vi "zlock_sendrecv.vi"(8 "error in (no error)":errorcluster, 10 "parts":string[](array[string]), 11 "socket in":T1) -> (0 "error out":errorcluster, 2 "reply":string, 3 "socket out":T1)   [LabVIEW 2010]
uses:
  <userlib>/BIAS2/subvis/zlock/zlock.ctl
  <vilib>/addons/zeromq/zmq_context.lvclass
  <vilib>/addons/zeromq/socket_type.ctl
  <vilib>/addons/zeromq/zmq_socket.lvclass
  <vilib>/addons/zeromq/zeromq.lvlib
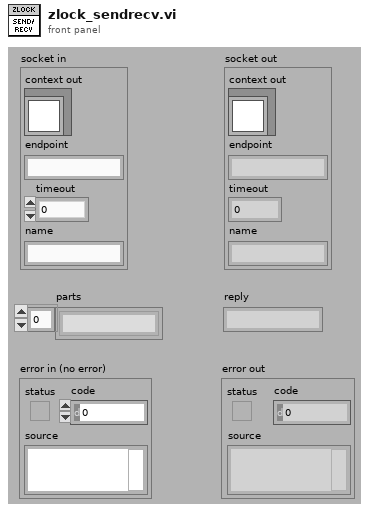
[diagram p1: front panel]
types:
  T1 = typedef "zlock.ctl" = cluster{"context out":refnum<class "zmq_context.lvclass">, "endpoint":string, "timeout":u32, "name":string}
  T2 = typedef "zeromq.lvlib/socket_type.ctl" = enum8{"ZMQ_PAIR", "ZMQ_PUB", "ZMQ_SUB", "ZMQ_REQ", "ZMQ_REP", "ZMQ_DEALER", "ZMQ_ROUTER", "ZMQ_PULL", "ZMQ_PUSH", "ZMQ_XPUB", "ZMQ_XSUB"}
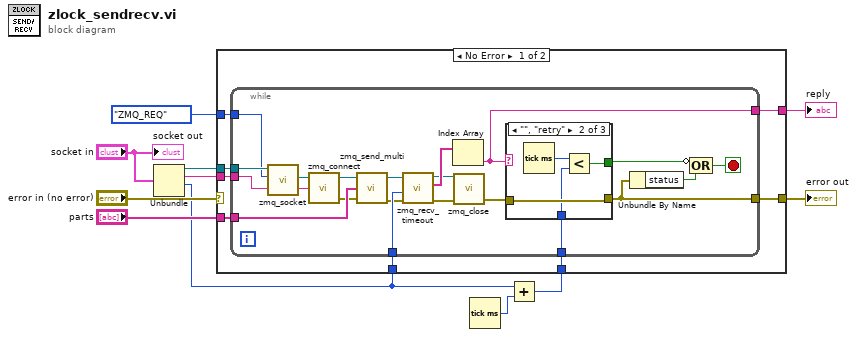
[diagram p0: block diagram]
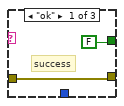
[diagram p2: hidden frame]
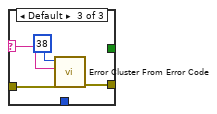
[diagram p3: hidden frame]
diagram:
  n1 = Unbundle("socket in") -> ("context out"=w5:refnum<class "zmq_context.lvclass">, "endpoint"=w4:string, "timeout"=w3:u32)  [unwired: 1 out]
  n2 = Tick Count (ms)() -> (millisecond timer value=w7:u32)
  n3 = Add(x=w3, y=w7) -> (x+y=w6:u32)
  n4 = case shown="No Error" "error in (no error)" {
    selector: "error in (no error)" -> [_ w50]
    tunnel: [w19 w50] -> w10
    tunnel: "parts" -> [w17 _]
    tunnel: [w18 _] -> w8
    tunnel: w6 -> [w16 _]
    tunnel: w3 -> [w15 _]
    tunnel: w5 -> [w14 _]
    tunnel: w4 -> [w13 _]
    tunnel: socket_type."ZMQ_REQ" ("socket type") -> [w12 _]
    frame No Error {
      n5 = while {
        tunnel: [w36] -> w19
        tunnel: [w38] -> w18
        tunnel: w17 -> [w37]
        tunnel: w16 -> [w32]
        tunnel: w15 -> [w31]
        tunnel: w14 -> [w30]
        tunnel: w13 -> [w28]
        tunnel: w12 -> [w20]
        stop <- w33 stop-if-true
        n6 = call <vilib>:"zmq_socket.vi"("socket type"=w20, "context in"=w30) -> ("socket out"=w27:refnum<class "zmq_socket.lvclass">)  [unwired: 3 in, 2 out]
        n7 = call <vilib>:"zmq_connect.vi"("endpoint"=w28, "socket in"=w27) -> ("error out"=w24:errorcluster, "socket out"=w29:refnum<class "zmq_socket.lvclass">)  [unwired: 2 in]
        n8 = call <vilib>:"zmq_send_multi.vi"("error in"=w24, "parts"=w37, "socket in"=w29) -> ("error out"=w25:errorcluster, "socket out"=w26:refnum<class "zmq_socket.lvclass">)  [unwired: 1 in]
        n9 = call <vilib>:"zmq_recv_timeout.vi"("error in"=w25, "timeout (ms)"=w31, "socket in"=w26) -> ("error out"=w23:errorcluster, "parts"=w39:string[], "socket out"=w22:refnum<class "zmq_socket.lvclass">)  [unwired: 1 in, 1 out]
        n10 = Index Array(array=w39) -> (element=w38:string)  [unwired: 1 in]
        n11 = call <vilib>:"zmq_close.vi"("error in"=w23, "socket"=w22) -> ("error out"=w21:errorcluster)  [unwired: 3 in]
        n12 = case shown="\"\", \"retry\"" w38 {
          selector: w38 -> [_ _ w48]
          tunnel: w21 -> [w41 w45 w49]
          tunnel: [w41 w45 w46] -> w36
          tunnel: [FALSE w42 _] -> w35
          tunnel: w32 -> [_ w43 _]
          frame "ok" {
            # "success"
          }
          frame "", "retry" {
            n13 = Tick Count (ms)() -> (millisecond timer value=w44:u32)
            n14 = Less?(x=w44, y=w43) -> (x < y?=w42:bool)
          }
          frame Default {
            n15 = call <vilib>:"Error Cluster From Error Code.vi"("error in (no error)"=w49, "error message (\"\")"=w48, "error code (0)"=38) -> ("error out"=w46:errorcluster)  [unwired: 6 in]
          }
        }
        n16 = Unbundle By Name(w36) -> ("status"=w34:bool)
        n17 = Compound Arithmetic op=OR(invert w35, w34) -> (w33:bool)
      }
    }
    frame Error {
    }
  }
  "error out" <- w10
  "reply" <- w8
  "socket out" <- "socket in"
